vi "Test.vi"() -> ()   [LabVIEW 2021]
uses:
  Example/String Indicator Event/String Indicator Event/String Indicator Event.lvclass
  C:/git/jettl/src/Actor/Msg/Msg.lvclass
  jettl/jettl.lvlib
panel:
  out "error out":errorcluster
  in  "Button":bool
  out "String Indicator":string
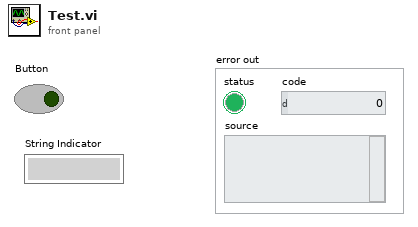
[diagram p1: front panel]
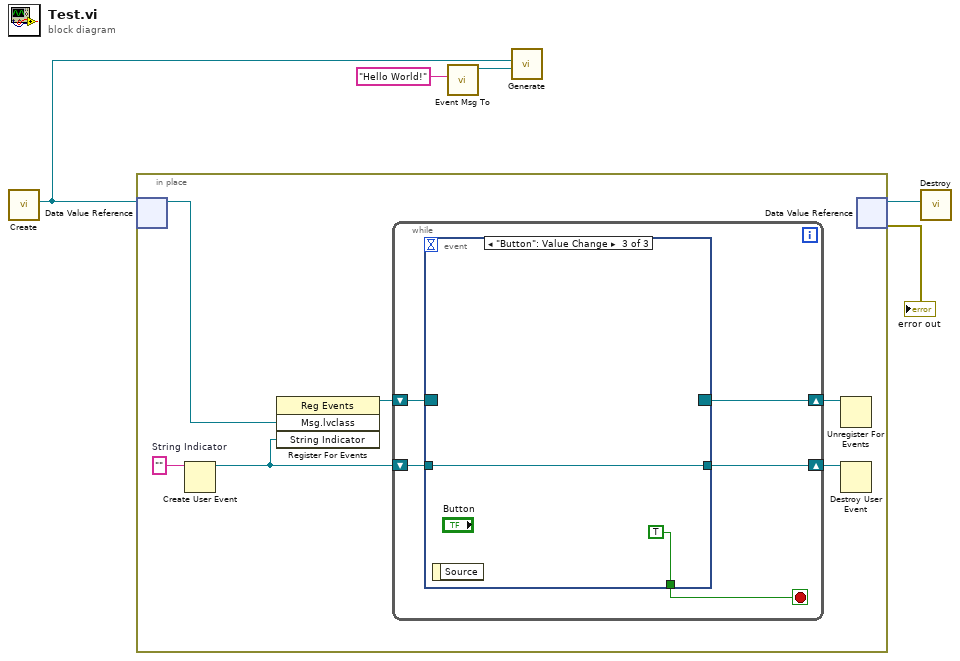
[diagram p0: block diagram]
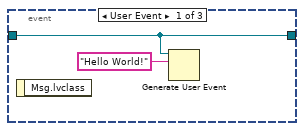
[diagram p2: hidden frame]
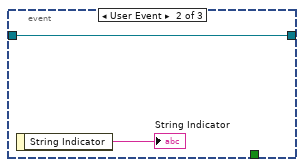
[diagram p3: hidden frame]
diagram:
  n1 = call "Create.vi"() -> ("Event"=w3:refnum<data-value>)  [unwired: 10 in, 1 out]
  n2 = in-place {
    w9 = ""  # String Indicator
    n3 = in-place-dvr #1(w3) -> (w6:refnum<user-event>)  [unwired: 1 out]
    n4 = Create User Event(user event datatype=w9) -> (user event=w8:refnum<user-event>)  [unwired: 1 in, 1 out]
    n5 = register-events(w6, w8) -> (reference out=w11:refnum<event-registration>)  [unwired: 2 in, 1 out]
    n6 = while {
      shift-right: [w15] -> w10
      shift-left: w11 -> [w16]
      shift-right: [w12] -> w7
      shift-left: w8 -> [w14]
      stop <- w13 stop-if-true
      n7 = event shown="[2] \"Button\": Value Change" {
        selector: w16 -> [_ _ _]
        dyn-events: [_ _ _] -> w15
        timeout: _ -> [_ _ _]
        tunnel: w14 -> [w18 w19 w21]
        tunnel: [_ _ TRUE] -> w13
        tunnel: [w18 w19 w21] -> w12
        event User Event {
          n8 = event-data() -> ()  [unwired: 1 in, 1 out]
          n9 = Generate User Event(user event=w18, event data cluster="Hello World!" ("event data")) -> ()  [unwired: 2 in, 2 out]
        }
        event User Event {
          n10 = event-data() -> ("String Indicator"=→"String Indicator":string)  [unwired: 1 in]
        }
        event "Button": Value Change {
          n11 = event-data() -> ()  [unwired: 1 in, 1 out]
        }
      }
    }
    n12 = Unregister For Events(event registration refnum=w10) -> ()  [unwired: 1 in, 1 out]
    n13 = Destroy User Event(user event=w7) -> ()  [unwired: 1 in, 1 out]
    n14 = in-place-dvr #1() -> (w5:refnum<data-value>, →"error out":errorcluster)  [unwired: 1 in]
  }
  n15 = call "Event Msg To.vi"("String Indicator"="Hello World!") -> ("String Indicator Event out"=w2:refnum<class "String Indicator Event.lvclass">)  [unwired: 10 in]
  n16 = call "Generate.vi"("Msg"=w2, "Event"=w3) -> ()  [unwired: 9 in, 1 out]
  n17 = call "Destroy.vi"("Event"=w5) -> ()  [unwired: 10 in, 1 out]
